vi "Replace Strings in File.vi"(6 "Use RegEx? (F)":bool, 8 "error in":errorcluster, 9 "Replace Strings":string[](array[string]), 10 "Search Strings":string[](array[string]), 11 "File Path":path) -> (0 "error out":errorcluster)   [LabVIEW 2020, in "ADAS_IO_Template_MDO.lvclass"]
uses:
  ADAS_IO_Template_MDO.lvclass
  ADAS_IO_Template_MDO.lvclass/ADAS_IO_Template_MDO.ctl
panel:
  out "# Replacements":i32
  out "DEBUG Output":string
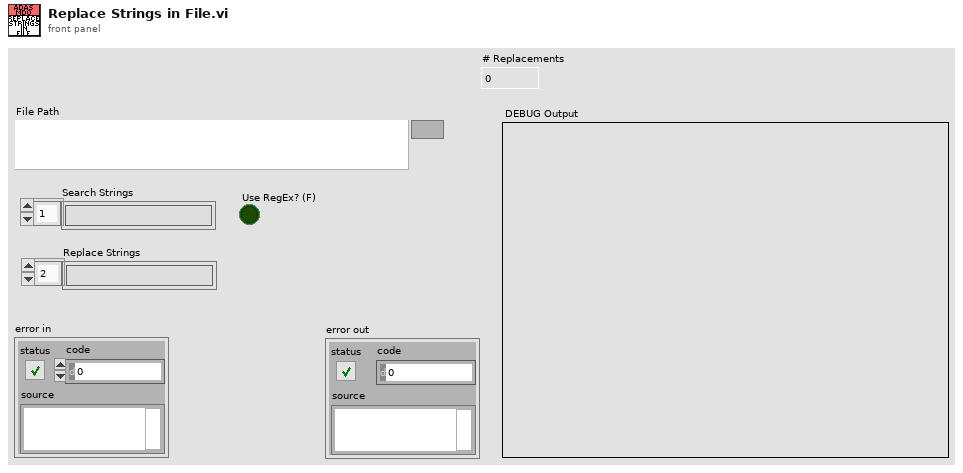
[diagram p1: front panel]
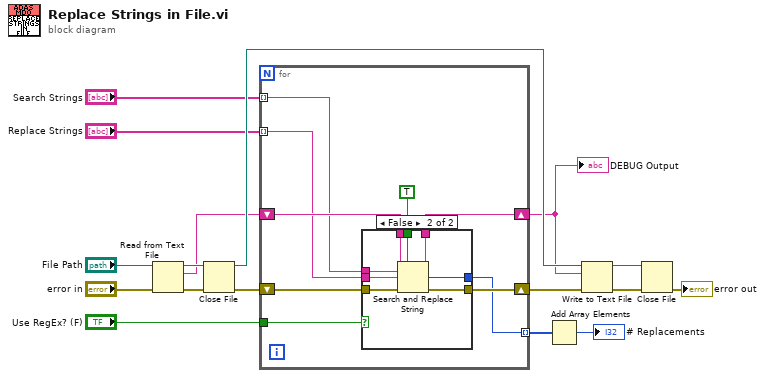
[diagram p0: block diagram]
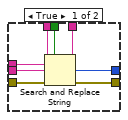
[diagram p2: hidden frame]
diagram:
  n1 = Read from Text File(file (use dialog)="File Path", error in="error in") -> (refnum out=w16:refnum<file>, text=w12:string, error out=w17:errorcluster)  [unwired: 2 in, 1 out]
  n2 = Close File(refnum=w16, error in=w17) -> (path=w14:path, error out=w15:errorcluster)
  n3 = for {
    shift-right: [w25] -> w13
    shift-left: w15 -> [w26]
    shift-right: [w23] -> w11
    shift-left: w12 -> [w24]
    tunnel: "Search Strings" -> [w21] mode=indexing
    tunnel: "Replace Strings" -> [w20] mode=indexing
    tunnel: "Use RegEx? (F)" -> [w19]
    tunnel: [w18] -> w2 mode=indexing
    n4 = case shown="False" w19 {
      tunnel: w26 -> [w34 w42]
      tunnel: [w33 w41] -> w25
      tunnel: w24 -> [w32 w40]
      tunnel: [w31 w39] -> w23
      tunnel: TRUE ("replace all? (F)") -> [w30 w38]
      tunnel: w21 -> [w29 w37]
      tunnel: w20 -> [w28 w36]
      tunnel: [w27 w35] -> w18
      frame True {
        n5 = Search and Replace String(replace all?=w30, input string=w32, search string=w29, replace string=w28, error in=w34) -> (result string=w31:string, number of replacements=w27:i32, error out=w33:errorcluster)  [unwired: 3 in, 1 out]
      }
      frame False {
        n6 = Search and Replace String(replace all?=w38, input string=w40, search string=w37, replace string=w36, error in=w42) -> (result string=w39:string, number of replacements=w35:i32, error out=w41:errorcluster)  [unwired: 3 in, 1 out]
      }
    }
  }
  "DEBUG Output" <- w11
  n7 = Add Array Elements(numeric array=w2) -> (sum=→"# Replacements":i32)
  n8 = Write to Text File(file (use dialog)=w14, text=w11, error in=w13) -> (refnum out=w9:refnum<file>, error out=w10:errorcluster)  [unwired: 1 in, 1 out]
  n9 = Close File(refnum=w9, error in=w10) -> (error out=→"error out":errorcluster)  [unwired: 1 out]
